vi "VI_caller.vi"(7 "VI_mostrar":i32, 8 "error in (no error)":errorcluster, 9 "SubPnl Refnum":refnum<vi>, 10 "path":path, 11 "VI_Action":T1=enum."Insert VI") -> (0 "error out":errorcluster, 2 "VI_Out_Array":refnum<vi>[](array[refnum]))   [LabVIEW 2026]
uses:
  Control/VI_Caller/Enum_VICaller.ctl
  Control/Ctrl_Array_Enc_Out.ctl
  Control/Ctr_Enc_Values.ctl
  Control/Ctrl_datos6motores_final.ctl
  Control/Ctrl_Motores_Valores.ctl
  Control/Ctrl_Errores.ctl
  Control/Ctrl_GuiEvent.ctl
  Control/Ctrl_ControlPIDEvent.ctl
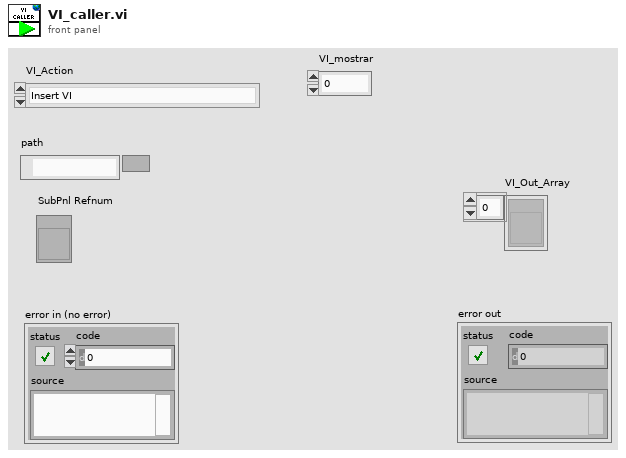
[diagram p1: front panel]
types:
  T1 = typedef "Enum_VICaller.ctl" = enum16{"Start", "Insert VI", "Stop"}
  T2 = typedef "Ctrl_GuiEvent.ctl" = enum16{"Set Ref", "Update Enc", "Stop", "Get Ref"}
  T3 = typedef "Ctrl_Array_Enc_Out.ctl" = T4[]
  T4 = typedef "Ctr_Enc_Values.ctl" = cluster{"Datos6_Motores":T5, "Errores":T7, "new_data?":bool}
  T5 = typedef "Ctrl_datos6motores_final.ctl" = cluster{"M_cadera":T6, "M_hombro":T6, "M_codo":T6, "M_antebrazo":T6, "M_muneca":T6, "M_gripper":T6}
  T6 = typedef "Ctrl_Motores_Valores.ctl" = cluster{"Pasos":i32, "Vueltas":i16, "Velocidad":dbl, "Reserva1":u8, "Reserva2":u8}
  T7 = typedef "Ctrl_Errores.ctl" = cluster{"Contador_correcto":u32, "Contador_errores":u32, "Edo_conex":u32}
  T8 = typedef "Ctrl_ControlPIDEvent.ctl" = enum16{"Set Ref", "Update Enc", "Stop", "Get Ref"}
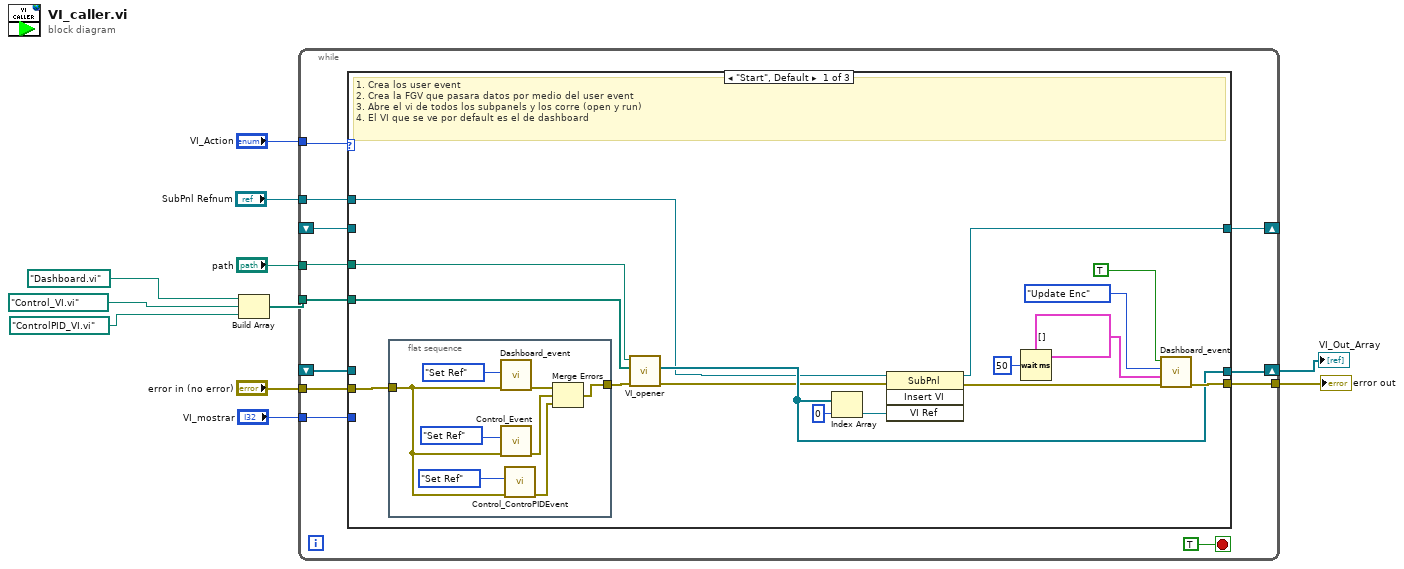
[diagram p0: block diagram]
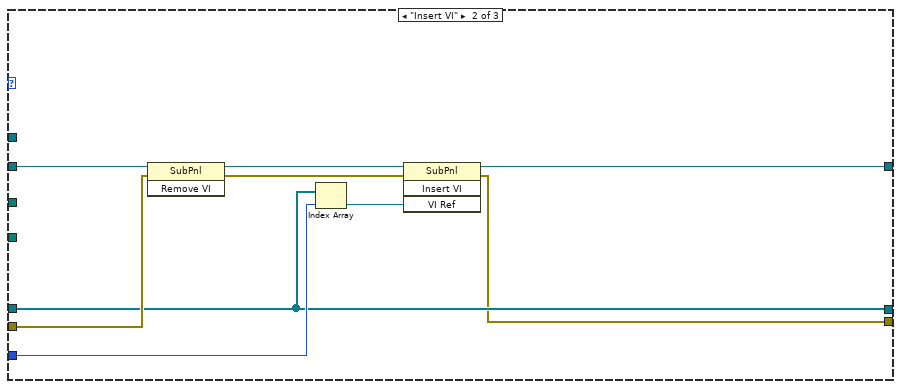
[diagram p2: hidden frame]
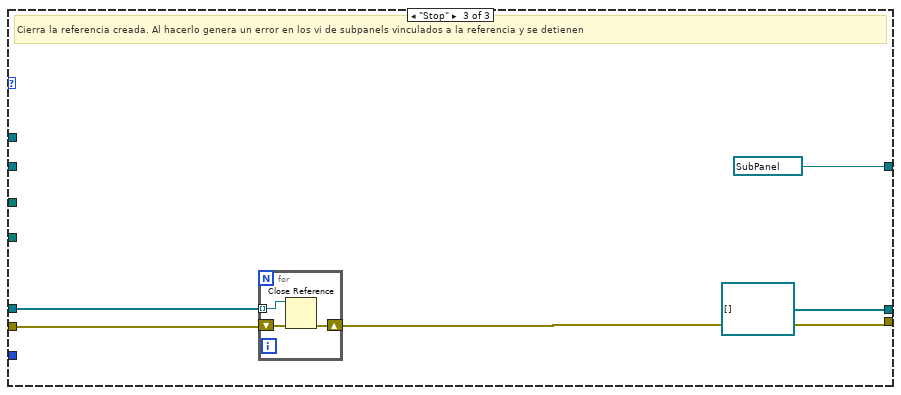
[diagram p3: hidden frame]
diagram:
  n1 = Build Array(path "Dashboard.vi" ("name or relative path"), path "Control_VI.vi" ("element"), path "ControlPID_VI.vi" ("element")) -> (w5:path[])
  n2 = while {
    tunnel: "path" -> [w23]
    tunnel: w5 -> [w20]
    tunnel: "VI_Action" -> [w19]
    shift-right: [w18] -> w7
    shift-left: _ -> [w17]
    shift-right: [w14] -> _
    shift-left: _ -> [w15]
    tunnel: "VI_mostrar" -> [w13]
    tunnel: "error in (no error)" -> [w22]
    tunnel: [w21] -> w9
    tunnel: "SubPnl Refnum" -> [w12]
    stop <- TRUE stop-if-true
    n3 = case shown="\"Start\", Default" w19 {
      tunnel: w20 -> [w28 _ _]
      tunnel: w23 -> [w29 _ _]
      tunnel: w22 -> [w38 w55 w61]
      tunnel: [w35 w50 w60] -> w21
      tunnel: [w27 w53 refnum<vi>[] []] -> w18
      tunnel: w17 -> [_ w53 w59]
      tunnel: w15 -> [_ w56 _]
      tunnel: [w32 w51 refnum<vi> refnum ("SubPnl Refnum")] -> w14
      tunnel: w13 -> [_ w54 _]
      tunnel: w12 -> [w25 _ _]
      frame "Start", Default {
        # "1. Crea los user event\n2. Crea la FGV que pasara datos por medio del user event\n3. Abre el vi de todos los subpanels y los corre (open y run)\n4. El VI que se ve por default es el de dashboard"
        n4 = flat-sequence {
          tunnel: w38 -> [w42]
          tunnel: [w46] -> w30
          frame #0 {
            n5 = call "Dashboard_event.vi"("error in"=w42, "Estado"=Ctrl_GuiEvent."Set Ref") -> ("error out"=w47:errorcluster)  [unwired: 8 in, 1 out]
            n6 = call "Control_Event.vi"("error in"=w42, "Estado"=Ctrl_GuiEvent."Set Ref") -> ("error out"=w45:errorcluster)  [unwired: 8 in, 1 out]
            n7 = call "Control_ControPIDEvent.vi"("error in"=w42, "Estado"=Ctrl_ControlPIDEvent."Set Ref") -> ("error out"=w40:errorcluster)  [unwired: 8 in, 1 out]
            n8 = Merge Errors(w47, w45, w40) -> (w46:errorcluster)
          }
        }
        n9 = call "VI_opener.vi"("error in (no error)"=w30, "vi_array_in"=w28, "path"=w29) -> ("error out"=w24:errorcluster, "vi_array_out"=w27:refnum<vi>[])  [unwired: 7 in]
        n10 = Index Array(array=w27, index=0) -> (element=w31:refnum<vi>)
        n11 = invoke on="Invoke Node" class="SubPnl" method="Insert VI"(reference=w25, error in=w24, "VI Ref"=w31) -> (reference out=w32:refnum<vi>, error out=w34:errorcluster)  [unwired: 1 in, 2 out]
        n12 = Wait (ms)(milliseconds to wait=u32 50) -> ()  [unwired: 1 out]
        n13 = call "Dashboard_event.vi"("error in"=w34, "array_enc_in"=T3 [], "Estado"=Ctrl_GuiEvent."Update Enc", "New_data?"=TRUE) -> ("error out"=w35:errorcluster)  [unwired: 6 in, 1 out]
      }
      frame "Insert VI" {
        n14 = invoke on="Invoke Node" class="SubPnl" method="Remove VI"(reference=w56, error in=w55) -> (reference out=w49:refnum<vi>, error out=w48:errorcluster)  [unwired: 1 in, 1 out]
        n15 = Index Array(array=w53, index=w54) -> (element=w52:refnum<vi>)
        n16 = invoke on="Invoke Node" class="SubPnl" method="Insert VI"(reference=w49, error in=w48, "VI Ref"=w52) -> (reference out=w51:refnum<vi>, error out=w50:errorcluster)  [unwired: 1 in, 2 out]
      }
      frame "Stop" {
        # "Cierra la referencia creada. Al hacerlo genera un error en los vi de subpanels vinculados a la referencia y se detienen"
        n17 = for {
          tunnel: w59 -> [w62] mode=indexing
          shift-right: [w63] -> w60
          shift-left: w61 -> [w64]
          n18 = Close Reference(reference=w62, error in (no error)=w64) -> (error out=w63:errorcluster)
        }
      }
    }
  }
  "error out" <- w9
  "VI_Out_Array" <- w7
